vi "Write Results Queue Table.vi"(8 "error in (no error)":errorcluster, 10 "Results Queue Table":variant, 11 "TestStand Controller in":refnum<class "Controller API.lvclass">) -> (0 "error out":errorcluster, 3 "TestStand Controller out":refnum<class "Controller API.lvclass">)   [LabVIEW 2017, in "Controller API.lvlib" / "Controller API.lvclass"]
uses:
  Controller API.lvclass
  Controller API.lvclass/Controller API.ctl
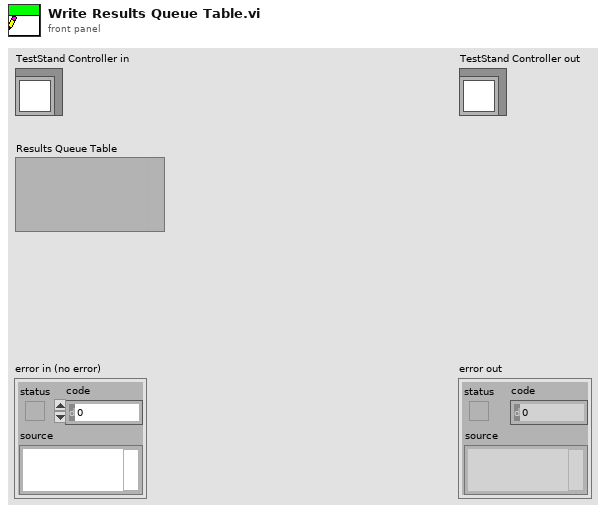
[diagram p1: front panel]
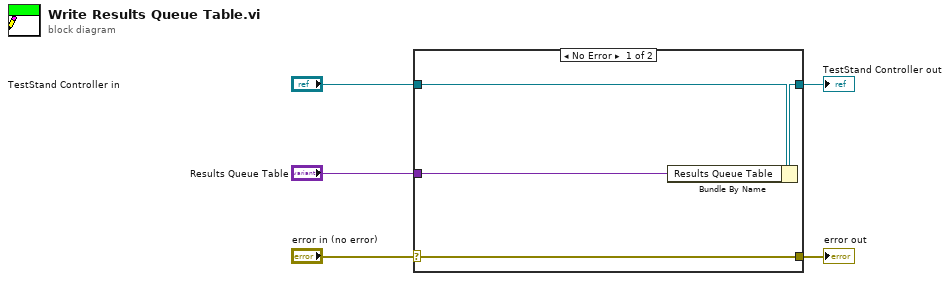
[diagram p0: block diagram]
diagram:
  n1 = case shown="No Error" "error in (no error)" {
    selector: "error in (no error)" -> [w9 w10]
    tunnel: [w9 w10] -> w4
    tunnel: [w7 w11] -> w2
    tunnel: "TestStand Controller in" -> [w8 w11]
    tunnel: "Results Queue Table" -> [w6 _]
    frame No Error {
      n2 = Bundle By Name(cluster=w8, "Results Queue Table"=w6) -> (w7:refnum<class "Controller API.lvclass">)
    }
    frame Error {
    }
  }
  "error out" <- w4
  "TestStand Controller out" <- w2
